vi "Insight_Diagnostic_PowerLevel.vi"(8 "error in (no error)":errorcluster, 11 "telnet connection":T1) -> (0 "error out":errorcluster, 1 "response data":string, 3 "telnet  connection out":T1)   [LabVIEW 2015]
doc: "Insight Photonic Solutions\n\nThis VI performs a power-leveling oepration on the laser sweep profile. This is a Diagnostic Mode function only. For best performance, power-leveling should be performed during sweep calibration.\n\nver 1.0 - original release\nver 1.1 - added data response buffer as an output"
uses:
  Telnet Session.ctl
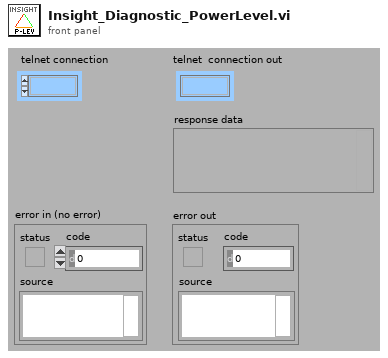
[diagram p1: front panel]
types:
  T1 = typedef "Telnet Session.ctl" = refnum<k1>
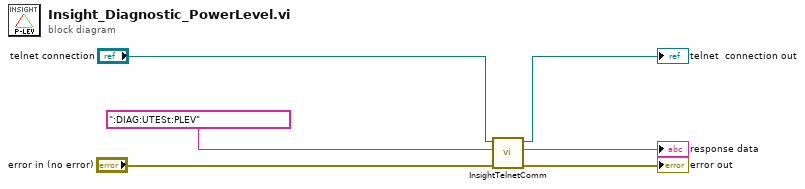
[diagram p0: block diagram]
diagram:
  n1 = call "InsightTelnetComm.vi"("error in"="error in (no error)", "write buffer (\"\")"=":DIAG:UTESt:PLEV" ("String"), "telnet connection"="telnet connection") -> ("error out"=→"error out":errorcluster, "response data"=→"response data":string, "telnet  connection out"=→"telnet  connection out":T1)  [unwired: 4 in]
